vi "CaptureFailure.vi"() -> ()   [LabVIEW 2014]
panel:
  in  "VISA resource name":refnum<visa-resource-name>="COM5"
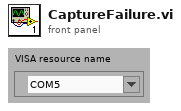
[diagram p1: front panel]
types:
  T1 = enum16{"Enter FAT", "Beeper Control", "LED Off", "LED On", "Image Mode", "Start Session", "Stop Session", "Change Buadrate", "Auto Exposure", "Set Manual Exposure", "Read BT Address", "Store BT Address", "Pairing Command", "Query Paired Address", "Pairing Status", "Un-Pairing", "Set Illumination", "Trigger", "Set Defaults", "Imager Time To Decode Test", "Battery Off", "Battery Charge Control", "Read Battery Voltage", "Read Battery Temperature", "Software Version", "StoreFeatureSet", "ReadFeatureSet", "Store Model Number", "Read Model Number", "Store Manufacturing Date", "Read Manufacturing Date", "Store Service Date", "Read Service Date", "Store Serial Number", "Read Serial Number", "Exit FAT", "Read GUID", "Cable Auto ID", "Store RSM 627", "Read RSM 627", "Hall Effect switch", "Store GUID "}
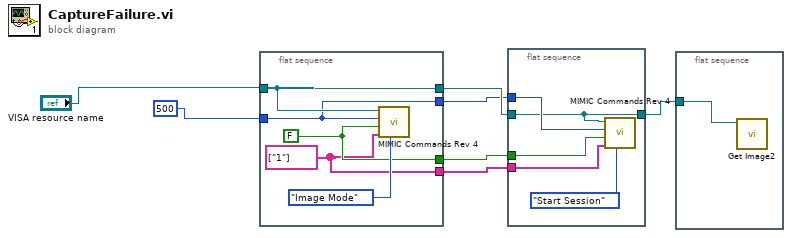
[diagram p0: block diagram]
diagram:
  n1 = flat-sequence {
    tunnel: "VISA resource name" -> [w11]
    tunnel: [w11] -> w6
    tunnel: u32 500 ("wait (ms)") -> [w10]
    tunnel: [w10] -> w4
    tunnel: [w9] -> w3
    tunnel: [w8] -> w2
    frame #0 {
      w8 = string[] ["1"] ("Input String Data Array")
      w9 = FALSE ("HWHSflag")
      n2 = call "MIMIC Commands Rev 4.vi"("MIMIC HOST COMMAND"=T1."Image Mode", "Input String Data Array"=w8, "HWHSflag"=w9, "wait (ms)"=w10, "VISA resource name"=w11) -> ()  [unwired: 4 in, 3 out]
    }
  }
  n3 = flat-sequence {
    tunnel: w2 -> [w16]
    tunnel: w3 -> [w15]
    tunnel: w4 -> [w14]
    tunnel: w6 -> [w13]
    tunnel: [w13] -> w7
    frame #0 {
      n4 = call "MIMIC Commands Rev 4.vi"("MIMIC HOST COMMAND"=T1."Start Session", "Input String Data Array"=w16, "HWHSflag"=w15, "wait (ms)"=w14, "VISA resource name"=w13) -> ()  [unwired: 4 in, 3 out]
    }
  }
  n5 = flat-sequence {
    tunnel: w7 -> [w18]
    frame #0 {
      n6 = call "Get Image2.vi"("VISA resource name"=w18) -> ()  [unwired: 9 in, 2 out]
    }
  }
